vi "Connect.vi"(8 "error in (no error)":errorcluster, 11 "Analog-Output in":refnum<class "Analog-Output.lvclass">) -> (0 "error out":errorcluster, 3 "Analog-Output out":refnum<class "Analog-Output.lvclass">)   [LabVIEW 2019, in "Analog-Output.lvlib" / "Analog-Output.lvclass"]
uses:
  Library/Analog-Output.lvclass
  builds/Instruments/Instruments.lvlibp/Library/Instruments.lvclass
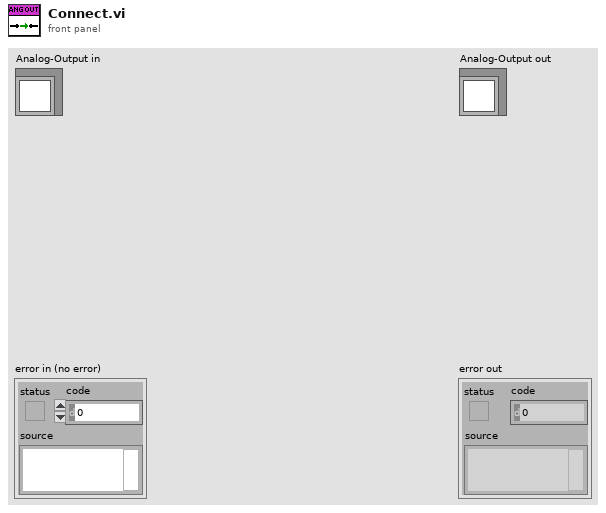
[diagram p1: front panel]
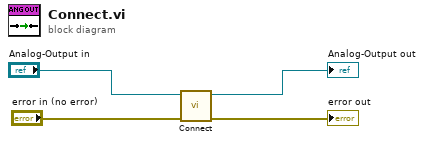
[diagram p0: block diagram]
diagram:
  n1 = call-parent "Connect.vi"("error in (no error)"="error in (no error)", "Instruments in"="Analog-Output in") -> ("error out"=→"error out":errorcluster, "Instruments out"=→"Analog-Output out":refnum<class "Analog-Output.lvclass">)  [unwired: 8 in]
